vi "Bandwidth and PSD.vi"() -> ()   [LabVIEW 2021]
uses:
  <vilib>/Analysis/4window.llb/windowTd.ctl
  <vilib>/measure/maspectr.llb/Power Spectrum and PSD Export Mode.ctl
  <vilib>/measure/madcrms.llb/Basic Averaged DC-RMS for 1 Chan.vi
  <vilib>/measure/maspectr.llb/FFT Power Spectrum and PSD for 1 Chan.vi
  <vilib>/measure/NI_MAPro.lvlib
  <vilib>/measure/NI_MABase.lvlib
  <vilib>/Analysis/NI_AALPro.lvlib
panel:
  out "Power Spectral density, 1-Hz increments":cluster{"f0":dbl, "df":dbl, "magnitude":dbl[]}(graph)={"f0"=0.0, "df"=1.0, "magnitude"=[1.109335647967048e-33, 2.4325025041771197e-33, 1.0255191767873154e-32, 4.930380657631324e-33, 1.0000000000000002, 1.0, 0.9999999999999997, 1.0, 1.0000000000000004, 9.757959141050148e-34, 9.553948047923692e-34, 5.969274723246312e-33, 2.938506871948269e-32, 2.6821270777514403e-33, 1.329230625297405e-32, 1.0728508311005761e-32, 1.4870028063416074e-32, 6.4094948549207215e-34, 1.0809859591856677e-32, 4.819344968658646e-33, 9.340247179796827e-35, 9.085985794341217e-34, 3.378543345641865e-32, 6.4094948549207215e-34, 1.7828256457994868e-32, 2.6821270777514403e-33, 6.47852018412756e-33, 6.4094948549207215e-34, 1.1125403953945083e-32, 1.6749343409861e-33, 6.026054830191291e-34, 1.7884764238144168e-33, 9.212416258784129e-33, 6.4094948549207215e-34, 6.794064546215964e-33, 3.944304526105059e-33, 2.749180254695226e-32, 2.6821270777514403e-33, 3.5104310282335025e-33, 3.442524071887468e-33, 5.205141354658209e-36, 3.696644609808852e-34, 1.0097419586828952e-32, 4.0389678347315806e-32, 1.0255191767873154e-32, 2.524354896707238e-33, 2.524354896707238e-33, 8.085824278515371e-33, 3.1554436208840474e-34, 2.8014611034788612e-34]}
  out "Expected Noise, \nRMS amplitude x sqrt(bandwidth)":dbl=2.2360679774997894 format="%.2f"
  out "Bandwidth, Hz":dbl=5.0 format="%.2f"
  out "RMS of any single frequency":dbl=0.9999999999999999 format="%.2f"
  out "peak-to-peak amplitude":dbl=8.988549547590623 format="%0.2p"
  out "RMS value":dbl=2.2360679774997894 format="%.2f"
  out "Waveform Graph 2":waveform(dbl)[](graph)=[{"t0"=timestamp(0 s since 1904-01-01), "dt"=0.01, "Y"=[-0.3913574979587439, -0.04109654050523885, 0.31174666373071286, 0.6450016785604361, 0.9377288657759673, 1.1715350996292688, 1.3317294745681585, 1.4082463888615269, 1.3962780033747964, 1.2965763357847397, 1.1154060085431263, 0.8641506196083991, 0.5585974691200124, 0.21794558526902796, -0.13640062125220098, -0.4821762750937618, -0.7976550202508859, -1.06301416691569, -1.2615802239805483, -1.3808765558052019, -1.4134073351198901, -1.3571285334204326, -1.2155763547965626, -0.9976450432237118, -0.7170280245033045, -0.39135749795874286, -0.04109654050523914, 0.3117466637307137, 0.645001678560436, 0.9377288657759677, 1.171535099629269, 1.3317294745681585, 1.4082463888615273, 1.396278003374796, 1.2965763357847404, 1.1154060085431254, 0.8641506196083998, 0.5585974691200113, 0.21794558526902852, -0.1364006212522021, -0.4821762750937615, -0.7976550202508866, -1.06301416691569, -1.2615802239805483, -1.380876555805202, -1.4134073351198895, -1.357128533420433, -1.2155763547965615, -0.9976450432237125, -0.7170280245033034, -0.3913574979587435, -0.041096540505238255, 0.31174666373071314, 0.6450016785604364, 0.9377288657759674, 1.1715350996292688, 1.3317294745681585, 1.4082463888615266, 1.3962780033747961, 1.2965763357847393, 1.1154060085431259, 0.8641506196083986, 0.5585974691200118, 0.2179455852690274, -0.13640062125220154, -0.48217627509376226, -0.7976550202508862, -1.0630141669156905, -1.2615802239805483, -1.380876555805202, -1.4134073351198897, -1.3571285334204326, -1.215576354796562, -0.9976450432237115, -0.7170280245033038, -0.3913574979587422, -0.04109654050523859, 0.31174666373071447, 0.6450016785604363, 0.9377288657759685, 1.171535099629269, 1.331729474568159, 1.408246388861527, 1.396278003374796, 1.29657633578474, 1.115406008543125, 0.8641506196083992, 0.5585974691200106, 0.21794558526902785, -0.13640062125220276, -0.48217627509376215, -0.7976550202508872, -1.0630141669156905, -1.2615802239805487, -1.3808765558052023, -1.4134073351198897, -1.357128533420433, -1.2155763547965615, -0.9976450432237121, -0.7170280245033029]}, {"t0"=timestamp(0 s since 1904-01-01), "dt"=0.01, "Y"=[1.2327120071235518, 1.3865659331503128, 1.4046931248673988, 1.2853191664499701, 1.0401292126751998, 0.6931241645574225, 0.2782712939327423, -0.16382070977218532, -0.5898768009986102, -0.9581916410299505, -1.2327120071235518, -1.3865659331503128, -1.404693124867399, -1.2853191664499704, -1.0401292126752, -0.6931241645574229, -0.2782712939327425, 0.16382070977218477, 0.5898768009986102, 0.9581916410299499, 1.2327120071235518, 1.3865659331503126, 1.404693124867399, 1.2853191664499706, 1.0401292126752, 0.6931241645574233, 0.2782712939327425, -0.16382070977218433, -0.5898768009986102, -0.9581916410299496, -1.2327120071235518, -1.3865659331503126, -1.404693124867399, -1.2853191664499708, -1.0401292126752, -0.6931241645574238, -0.2782712939327425, 0.16382070977218388, 0.5898768009986102, 0.9581916410299495, 1.2327120071235518, 1.3865659331503126, 1.404693124867399, 1.285319166449971, 1.0401292126752, 0.6931241645574241, 0.2782712939327425, -0.16382070977218355, -0.5898768009986102, -0.9581916410299492, -1.2327120071235518, -1.3865659331503126, -1.404693124867399, -1.2853191664499712, -1.0401292126752, -0.6931241645574245, -0.2782712939327425, 0.1638207097721831, 0.5898768009986102, 0.9581916410299489, 1.2327120071235518, 1.3865659331503126, 1.404693124867399, 1.2853191664499715, 1.0401292126752, 0.6931241645574249, 0.2782712939327425, -0.16382070977218266, -0.5898768009986102, -0.9581916410299485, -1.2327120071235518, -1.3865659331503124, -1.404693124867399, -1.2853191664499717, -1.0401292126752, -0.6931241645574253, -0.2782712939327425, 0.16382070977218222, 0.5898768009986102, 0.9581916410299481, 1.2327120071235518, 1.3865659331503122, 1.404693124867399, 1.2853191664499717, 1.0401292126752, 0.6931241645574256, 0.2782712939327425, -0.16382070977218166, -0.5898768009986102, -0.9581916410299476, -1.2327120071235518, -1.386565933150312, -1.404693124867399, -1.285319166449972, -1.0401292126752, -0.6931241645574261, -0.2782712939327425, 0.16382070977218122, 0.5898768009986102, 0.9581916410299472]}, {"t0"=timestamp(0 s since 1904-01-01), "dt"=0.01, "Y"=[0.19617291926721944, -0.33317670529192267, -0.815732651719518, -1.1837213713882344, -1.3854599422008302, -1.3926147814086218, -1.204181013107457, -0.8466236000721898, -0.37016041838290537, 0.15829069403422524, 0.6645103488788132, 1.0774014999996133, 1.3389748122419292, 1.412493091238751, 1.2876309131848693, 0.9819247999254648, 0.5383102665775769, 0.0190916560266694, -0.5028083208770485, -0.9540903633475389, -1.2713732496291903, -1.410095541237572, -1.3507741045679327, -1.1017404591104718, -0.697970640297354, -0.1961729192672209, 0.3331767052919208, 0.815732651719517, 1.1837213713882333, 1.3854599422008302, 1.392614781408622, 1.204181013107458, 0.8466236000721913, 0.3701604183829065, -0.15829069403422336, -0.6645103488788123, -1.0774014999996124, -1.338974812241929, -1.4124930912387514, -1.2876309131848702, -0.9819247999254661, -0.5383102665775782, -0.019091656026671067, 0.5028083208770476, 0.9540903633475379, 1.2713732496291903, 1.4100955412375722, 1.3507741045679336, 1.1017404591104731, 0.6979706402973552, 0.1961729192672227, -0.33317670529192, -0.8157326517195157, -1.1837213713882333, -1.3854599422008302, -1.3926147814086227, -1.204181013107459, -0.8466236000721924, -0.37016041838290825, 0.15829069403422225, 0.6645103488788108, 1.0774014999996115, 1.3389748122419283, 1.4124930912387514, 1.2876309131848709, 0.9819247999254671, 0.53831026657758, 0.019091656026672288, -0.5028083208770454, -0.954090363347537, -1.271373249629189, -1.4100955412375722, -1.3507741045679338, -1.101740459110474, -0.6979706402973569, -0.1961729192672239, 0.3331767052919177, 0.8157326517195147, 1.1837213713882315, 1.38545994220083, 1.3926147814086227, 1.20418101310746, 0.8466236000721941, 0.3701604183829098, -0.15829069403421991, -0.6645103488788094, -1.07740149999961, -1.3389748122419278, -1.4124930912387514, -1.2876309131848716, -0.9819247999254685, -0.5383102665775813, -0.01909165602667462, 0.5028083208770443, 0.954090363347535, 1.2713732496291887, 1.4100955412375715, 1.3507741045679345, 1.101740459110475, 0.6979706402973581]}, {"t0"=timestamp(0 s since 1904-01-01), "dt"=0.01, "Y"=[-0.3568822874108205, 0.25973775444651165, 0.8269177809507798, 1.23669740229236, 1.4110767496663785, 1.3168634301155613, 0.9719905622771319, 0.4421032808644515, -0.1719365452568553, -0.753248955776353, -1.1911835195995935, -1.4023811901944458, -1.3466413579152632, -1.0345738710281662, -0.5255794946462868, 0.08345678107340593, 0.6766074011001908, 1.1409685797549531, 1.388151072851838, 1.3711047074971905, 1.093074189362094, 0.6069814862771851, 0.005352348897163184, -0.5972955861244048, -1.0862507581849805, -1.3684425574105852, -1.3901569331967818, -1.1472606432487062, -0.68598799928521, -0.09414035559189138, 0.5156265183485822, 1.0272460011332187, 1.3433334243771684, 1.4037228445833376, 1.1969193835099463, 0.762287231058163, 0.18255683331173533, -0.4319225082721867, -0.9641871734190406, -1.3129227680284004, -1.4117489032022885, -1.2418544297849257, -0.835578063386038, -0.27025284261278215, 0.3465138973822649, 0.897323139426597, 1.2773306053315805, 1.4142034338670246, 1.2818884439748648, 0.9055712508370347, 0.3568822874108154, -0.2597377544465166, -0.8269177809507838, -1.236697402292363, -1.4110767496663785, -1.3168634301155597, -0.9719905622771279, -0.4421032808644467, 0.17193654525686042, 0.7532489557763575, 1.1911835195995961, 1.402381190194447, 1.3466413579152614, 1.034573871028163, 0.5255794946462821, -0.08345678107341148, -0.6766074011001949, -1.1409685797549567, -1.3881510728518385, -1.3711047074971894, -1.0930741893620906, -0.6069814862771802, -0.005352348897158299, 0.5972955861244099, 1.0862507581849832, 1.368442557410587, 1.3901569331967805, 1.1472606432487034, 0.6859879992852055, 0.09414035559188605, -0.5156265183485865, -1.0272460011332227, -1.3433334243771693, -1.4037228445833376, -1.1969193835099432, -0.7622872310581589, -0.18255683331173045, 0.4319225082721919, 0.9641871734190437, 1.3129227680284028, 1.4117489032022874, 1.2418544297849237, 0.8355780633860336, 0.27025284261277704, -0.34651389738226956, -0.8973231394266017, -1.2773306053315818, -1.4142034338670253, -1.2818884439748621, -0.905571250837031]}, {"t0"=timestamp(0 s since 1904-01-01), "dt"=0.01, "Y"=[-1.386593259696783, -1.0810883311168038, -0.5081365928534717, 0.1905213497323519, 0.8420468557763369, 1.2852612195211208, 1.4105191287590235, 1.1868334502012454, 0.6695410322626913, -0.013386891930725175, -0.6930030779105298, -1.2011795609971867, -1.4122002685574495, -1.273861496796076, -0.8203864096287029, -0.16395868515359058, 0.5330302275261013, 1.0981545832464383, 1.3916101665131753, 1.34079998661846, 0.9582938032397834, 0.33871853582886335, -0.36465117203676267, -0.9778110517121434, -1.3490735408353698, -1.3865932596967827, -1.0810883311168025, -0.5081365928534695, 0.19052134973235302, 0.8420468557763389, 1.285261219521121, 1.4105191287590235, 1.1868334502012445, 0.6695410322626894, -0.013386891930726286, -0.6930030779105318, -1.201179560997187, -1.4122002685574495, -1.2738614967960753, -0.8203864096287009, -0.16395868515358947, 0.5330302275261035, 1.0981545832464388, 1.3916101665131757, 1.3407999866184594, 0.9582938032397816, 0.33871853582886224, -0.3646511720367651, -0.9778110517121441, -1.349073540835371, -1.3865932596967823, -1.081088331116801, -0.5081365928534683, 0.19052134973235568, 0.8420468557763398, 1.2852612195211222, 1.4105191287590233, 1.186833450201243, 0.6695410322626882, -0.013386891930729172, -0.693003077910533, -1.2011795609971885, -1.4122002685574497, -1.273861496796074, -0.8203864096287, -0.1639586851535868, 0.5330302275261046, 1.0981545832464403, 1.391610166513176, 1.3407999866184583, 0.958293803239781, 0.3387185358288596, -0.3646511720367658, -0.9778110517121459, -1.349073540835371, -1.3865932596967816, -1.0810883311168005, -0.5081365928534659, 0.19052134973235635, 0.8420468557763418, 1.2852612195211224, 1.4105191287590229, 1.1868334502012428, 0.6695410322626858, -0.013386891930729838, -0.6930030779105352, -1.201179560997189, -1.4122002685574495, -1.2738614967960737, -0.8203864096286975, -0.16395868515358614, 0.5330302275261072, 1.098154583246441, 1.3916101665131762, 1.3407999866184583, 0.9582938032397786, 0.3387185358288589, -0.36465117203676856, -0.9778110517121466, -1.3490735408353713]}]
  in  "stop":bool
  in  "Number of frequencies":i32=5
  out "Waveform Graph":waveform(dbl)(graph)={"t0"=timestamp(0 s since 1904-01-01), "dt"=0.01, "Y"=[-0.7059481186755754, 0.19094211068285938, 1.2194883249759023, 2.173818225646883, 2.8455217416930525, 3.0741691324147515, 2.788329446429601, 2.0267388100828496, 0.9338452709991176, -0.26996045891806186, -1.3369822472117352, -2.048574564733931, -2.265962469978171, -1.9633158577664338, -1.234864825017524, -0.27387754380590595, 0.6720215810202387, 1.3590213618845537, 1.6052494955060264, 1.33512941599286, 0.5992994149763506, -0.4349581194016414, -1.5209561576366921, -2.3891729737207585, -2.8101937511458077, -2.649442069775909, -1.9008938055941607, -0.6917386304241342, 0.7433795993971986, 2.11290366713129, 3.1323256117840383, 3.587109684417544, 3.3803437386447315, 2.5543831321537604, 1.28168892065454, -0.17294435174547385, -1.510144902009403, -2.460679410179364, -2.8427193751862267, -2.5991490710642213, -1.8070966562515547, -0.6582235559369767, 0.5851638217854348, 1.6479045872468598, 2.3006569042182585, 2.4067070217331006, 1.9472874429103244, 1.0209293018294467, -0.18170399284912597, -1.4207513152342337, -2.457607558101038, -3.101665264510789, -3.243733486660455, -2.8702149118377767, -2.0568901829901045, -0.9458060569312159, 0.287805734009851, 1.4701736678983164, 2.4574719635100477, 3.1529207346945434, 3.5108088062345546, 3.529319681955585, 3.2367064955871543, 2.6764702171898405, 1.8965525896254527, 0.9454572231621283, -0.12465063331465676, -1.250557217169721, -2.350806252194871, -3.3234632810614215, -4.052272977994944, -4.422052958256639, -4.34104710516582, -3.7652201343718925, -2.7179506601262484, -1.2988052840695836, 0.3228774729339208, 1.930424075617652, 3.2951091999648456, 4.217567660374979, 4.566496589333983, 4.305749548451735, 3.5030631396251932, 2.3175757758870246, 0.9681085789850424, -0.3112704847469608, -1.3187159807673967, -1.9244758131793687, -2.0940986303453712, -1.889686817067325, -1.4490228640940799, -0.9476465626677469, -0.5530663011772792, -0.3822280604275077, -0.47262931589666235, -0.774187586234931, -1.163916355618318, -1.479836146360231, -1.5657272788016403, -1.3155105348484097]}
  in  "fundamental frequency":dbl=4.0
  in  "sampling info":cluster{"Fs":dbl, "#s":dbl}={"Fs"=100.0, "#s"=100.0} {"Fs" format="%#.6g"}
  # "INDIVIDUAL COMPONENTS:\nRMS amplitude: 1 unit;  Phase: random"
  # "SUM:"
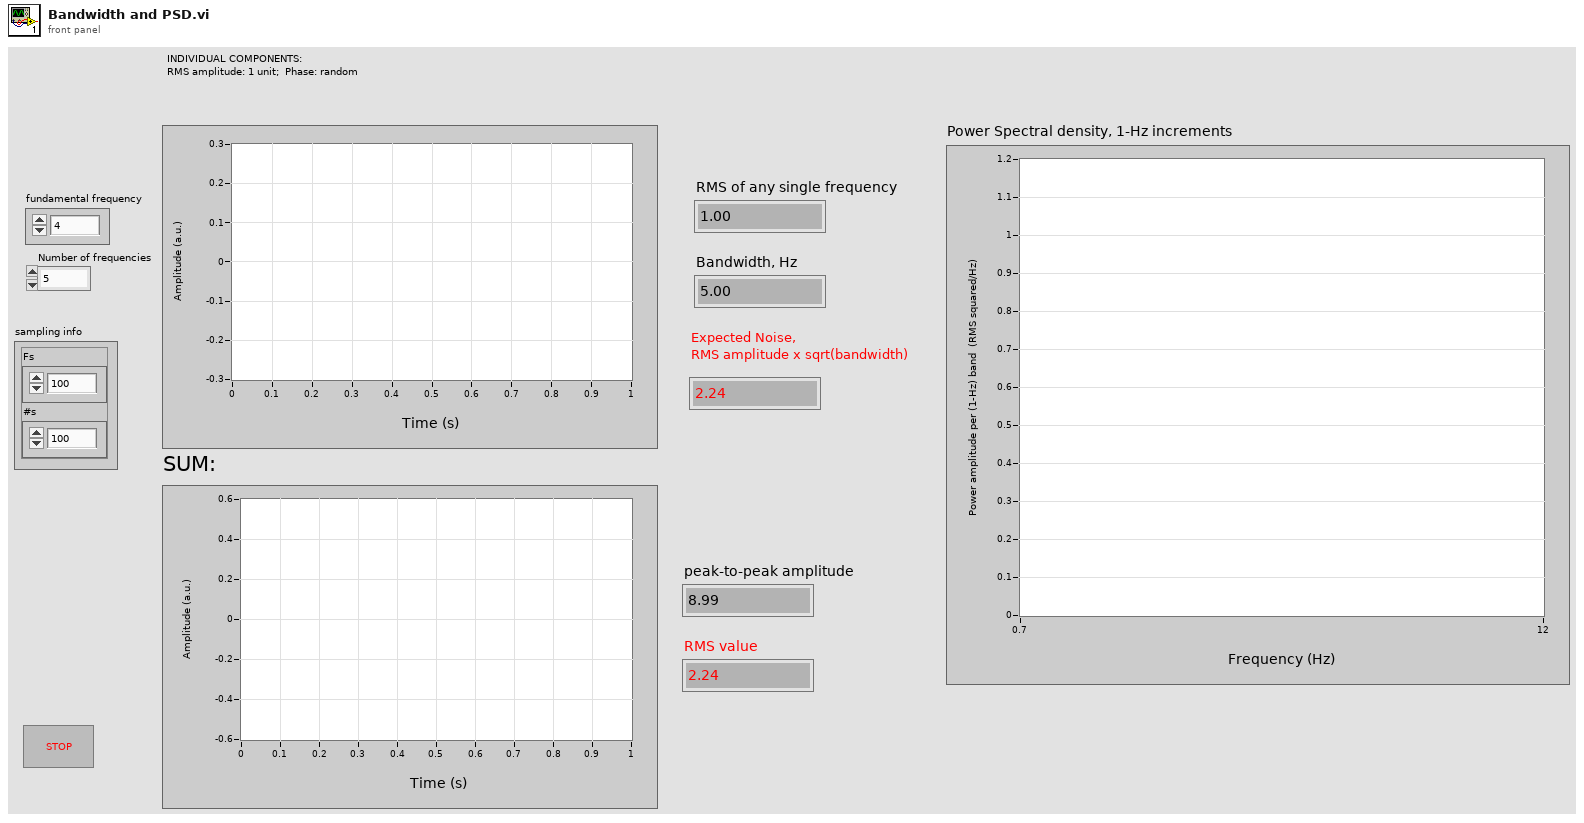
[diagram p1: front panel]
types:
  T1 = cluster{"averaging mode":enum16{"No averaging", "Vector averaging", "RMS averaging", "Peak hold"}, "weighting mode":enum16{"Linear", "Exponential"}, "number of averages":u32}
  T2 = typedef "NI_MAPro.lvlib/Power Spectrum and PSD Export Mode.ctl" = u16
  T3 = typedef "NI_AALPro.lvlib/windowTd.ctl" = u32
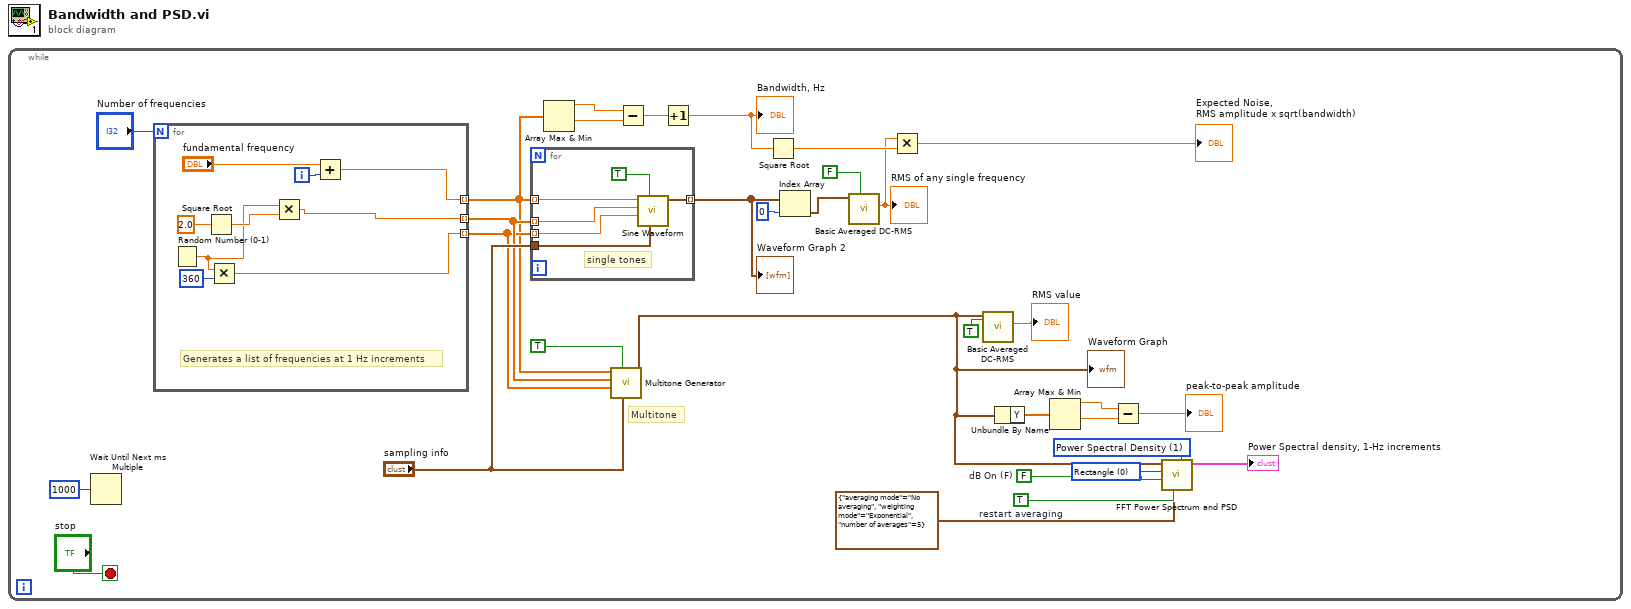
[diagram p0: block diagram]
diagram:
  n1 = while {
    stop <- "stop" stop-if-true
    w2 = T2 1 items=["Power Spectrum", "Power Spectral Density"] ("export mode")
    w5 = T3 0 items=["Rectangle"=0, "Hanning"=1, "Hamming"=2, "Blackman-Harris"=3, "Exact Blackman"=4, "Blackman"=5, "Flat Top"=6, "4 Term B-Harris "=7, "7 Term B-Harris"=8, "Low Sidelobe"=9, "Blackman Nuttall"=11, "Triangle"=30, "Bartlett-Hanning"=31, "Bohman"=32, "Parzen"=33, "Welch"=34, "Kaiser"=60, "Dolph-Chebyshev"=61, "Gaussian"=62] ("window")
    w6 = TRUE  # restart averaging
    w3 = FALSE  # dB On (F)
    # "Multitone"
    n2 = Wait Until Next ms Multiple(millisecond multiple=u32 1000) -> ()  [unwired: 1 out]
    n3 = for {
      N: "Number of frequencies" -> [_]
      tunnel: [w41] -> w26 mode=indexing
      tunnel: [w44] -> w16 mode=indexing
      tunnel: [w39] -> w27 mode=indexing
      i -> [w45]
      # "Generates a list of frequencies at 1 Hz increments"
      n4 = Random Number (0-1)() -> (number: 0 to 1=w40:dbl)
      n5 = Square Root(x=2.0) -> (sqrt(x)=w43:dbl)
      n6 = Multiply(x=w40, y=360) -> (x*y=w41:dbl)
      n7 = Multiply(x=w40, y=w43) -> (x*y=w39:dbl)
      n8 = Add(x="fundamental frequency", y=w45) -> (x+y=w44:dbl)
    }
    n9 = for {
      tunnel: "sampling info" -> [w38]
      tunnel: w16 -> [w37] mode=indexing
      tunnel: w27 -> [w36] mode=indexing
      tunnel: w26 -> [w35] mode=indexing
      tunnel: [w34] -> w20 mode=indexing
      # "single tones"
      n10 = call <vilib>:"Sine Waveform.vi"("sampling info"=w38, "reset signal"=TRUE, "phase"=w35, "amplitude"=w36, "frequency"=w37) -> ("signal out"=w34:waveform(dbl))  [unwired: 5 in, 1 out]
    }
    "Waveform Graph 2" <- w20
    n11 = Array Max & Min(array=w16) -> (max value=w11:dbl, min value=w10:dbl)  [unwired: 2 out]
    n12 = call <vilib>:"Multitone Generator.vi"("sampling info"="sampling info", "reset signal"=TRUE, "tone phases"=w26, "tone amplitudes"=w27, "tone frequencies"=w16) -> ("signal out"=w7:waveform(dbl))  [unwired: 3 in, 3 out]
    "Waveform Graph" <- w7
    n13 = Subtract(x=w11, y=w10) -> (x-y=w9:dbl)
    n14 = Increment(x=w9) -> (x+1=w8:dbl)
    "Bandwidth, Hz" <- w8
    n15 = Square Root(x=w8) -> (sqrt(x)=w14:dbl)
    n16 = Index Array(array=w20, index=0) -> (element=w17:waveform(dbl))
    n17 = call-poly <vilib>:"Basic Averaged DC-RMS.vi"("reset"=FALSE, "signal in"=w17) -> ("RMS value"=w12:dbl)  [unwired: 6 in, 3 out]
    "RMS of any single frequency" <- w12
    n18 = Multiply(x=w12, y=w14) -> (x*y=→"Expected Noise, \nRMS amplitude x sqrt(bandwidth)":dbl)
    n19 = call-poly <vilib>:"Basic Averaged DC-RMS.vi"("reset"=TRUE, "signal in"=w7) -> ("RMS value"=→"RMS value":dbl)  [unwired: 6 in, 3 out]
    n20 = Unbundle By Name(w7) -> ("Y"=w23:dbl[])
    n21 = Array Max & Min(array=w23) -> (max value=w22:dbl, min value=w21:dbl)  [unwired: 2 out]
    n22 = Subtract(x=w22, y=w21) -> (x-y=→"peak-to-peak amplitude":dbl)
    n23 = call-poly <vilib>:"FFT Power Spectrum and PSD.vi"("export mode"=w2, "averaging parameters"=T1 {"averaging mode"=enum."No averaging", "weighting mode"=enum."Exponential", "number of averages"=5}, "restart averaging (F)"=w6, "dB On (F)"=w3, "window"=w5, "time signal"=w7) -> ("Power Spectrum / PSD"=→"Power Spectral density, 1-Hz increments":cluster{"f0":dbl, "df":dbl, "magnitude":dbl[]})  [unwired: 2 in, 3 out]
  }
